vi "EX1 2.vi"() -> ()   [LabVIEW 2014]
panel:
  in  "문자열":string
  in  "수평 포인터 슬라이드":dbl(slide) scale=0.0..10.0
  in  "불리언":bool
  out "게이지":dbl(knob) scale=0.0..10.0
  out "온도계 2":dbl(slide) scale=0.0..100.0
  in  "온도계":dbl(slide) scale=0.0..100.0
  out "A4":dbl
  out "A3":dbl
  in  "A2":dbl
  in  "A":dbl
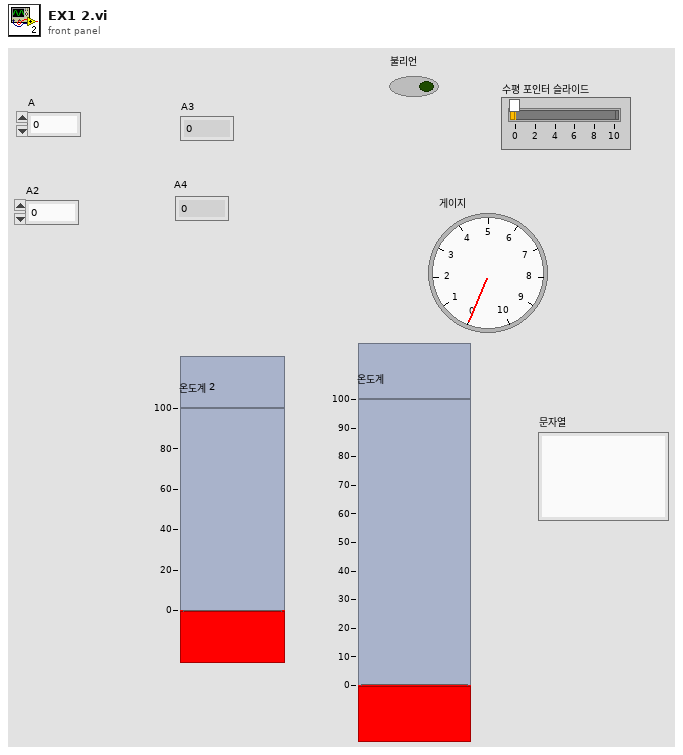
[diagram p1: front panel]
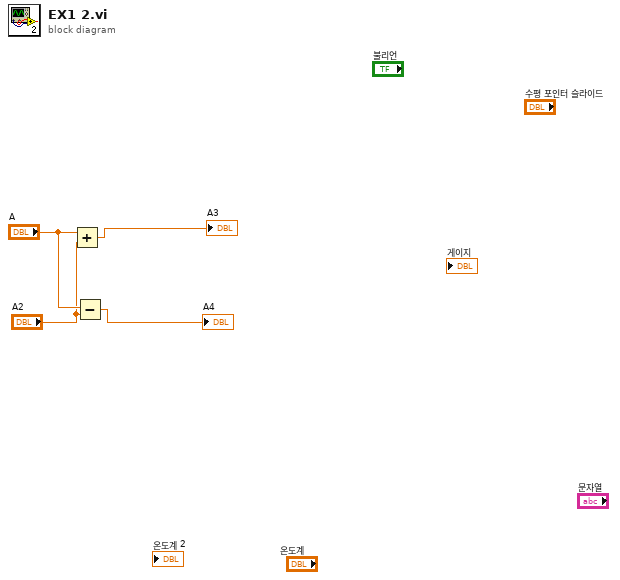
[diagram p0: block diagram]
diagram:
  n1 = Add(x="A", y="A2") -> (x+y=→"A3":dbl)
  n2 = Subtract(x="A", y="A2") -> (x-y=→"A4":dbl)
